vi "Listen for Connection.vi"(8 "error in (no error)":errorcluster, 11 "TCP Writer in":refnum<class "TCP Writer.lvclass">) -> (0 "error out":errorcluster, 2 "New Connection Made?":bool, 3 "TCP Writer out":refnum<class "TCP Writer.lvclass">)   [LabVIEW 2012, in "TCP Classes.lvlib" / "TCP Writer.lvclass"]
uses:
  TCP Writer.lvclass
  Class TCP Connection/TCP Connection.lvclass
  TCP Writer.lvclass/TCP Writer.ctl
  Common/Controls/Waveform Header with Enbl.ctl
  Common/Controls/Waveform Header.ctl
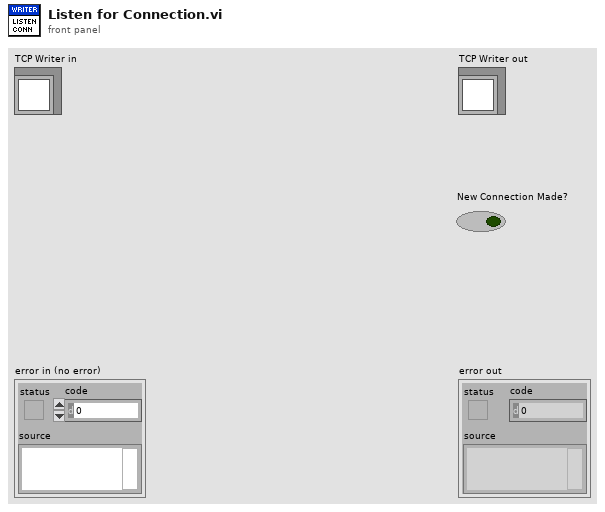
[diagram p1: front panel]
types:
  T1 = typedef "Waveform Header with Enbl.ctl" = cluster{"Send Wfm Hdr?":bool, "Wfm Header":T2}
  T2 = typedef "Waveform Header.ctl" = cluster{"dt":dbl, "attributes (str)":string[][]}
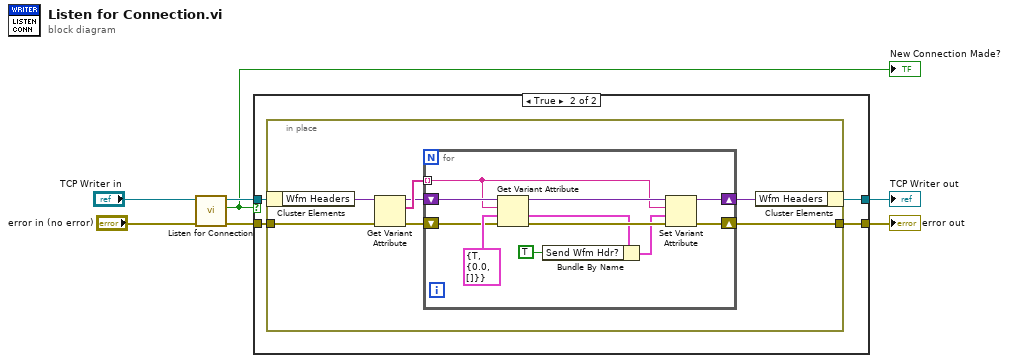
[diagram p0: block diagram]
diagram:
  n1 = call-parent "Listen for Connection.vi"("error in (no error)"="error in (no error)", "TCP Connection in"="TCP Writer in") -> ("error out"=w2:errorcluster, "New Connection Made?"=w3:bool, "TCP Connection out"=w5:refnum<class "TCP Writer.lvclass">)  [unwired: 7 in]
  "New Connection Made?" <- w3
  n2 = case shown="True" w3 {
    tunnel: w5 -> [w9 w13]
    tunnel: [w9 w12] -> w4
    tunnel: w2 -> [w8 w11]
    tunnel: [w8 w10] -> w1
    frame False {
    }
    frame True {
      n3 = in-place {
        in-place-border: w11 -> [w16]
        in-place-border: [w14] -> w10
        n4 = in-place-cluster #1(w13) -> ("Wfm Headers"=w19:variant)
        n5 = Get Variant Attribute(Variant=w19, error in=w16) -> (duplicate Variant=w17:variant, names=w18:string[], error out=w15:errorcluster)  [unwired: 2 in, 1 out]
        n6 = for {
          shift-right: [w29] -> w20
          shift-left: w17 -> [w31]
          tunnel: w18 -> [w28] mode=indexing
          shift-right: [w21] -> w14
          shift-left: w15 -> [w26]
          n7 = Get Variant Attribute(Variant=w31, name=w28, default value (empty Variant)=T1 {"Send Wfm Hdr?"=TRUE, "Wfm Header"={"dt"=0.0, "attributes (str)"=[]}} ("Wfm Header with Enbl"), error in=w26) -> (duplicate Variant=w30:variant, value=w23:T1, error out=w25:errorcluster)  [unwired: 1 out]
          n8 = Bundle By Name(cluster=w23, "Send Wfm Hdr?"=TRUE) -> (w22:T1)
          n9 = Set Variant Attribute(Variant=w30, name=w28, value=w22, error in=w25) -> (Variant out=w29:variant, error out=w21:errorcluster)  [unwired: 1 out]
        }
        n10 = in-place-cluster #1("Wfm Headers"=w20) -> (w12:refnum<class "TCP Writer.lvclass">)
      }
    }
  }
  "error out" <- w1
  "TCP Writer out" <- w4
